vi "MotorControl_PWM+AO.vi"() -> ()   [LabVIEW 2015]
uses:
  <vilib>/Platform/TimedLoop/XDataNode/timing_clust.ctl
  <vilib>/Platform/TimedLoop/XDataNode/nitl_modes.ctl
  <vilib>/Platform/TimedLoop/XDataNode/wakeup.ctl
  <vilib>/rvi/FXPMathLib/FxpDiv/subVIs/nifxpmath_Div_SimConfig.ctl
  <vilib>/rvi/Emulation/niFpgaGetClockAttributes.vi
  <vilib>/rvi/Emulation/niFpgaSctlEmulationGetInTimedLoop.vi
  <vilib>/rvi/Emulation/niFpgaEmulationReportErrorSimple.vi
  <vilib>/rvi/FXPMathLib/FxpDiv/simVIs/DllFxpDivTemp_sub.vi
  GVEncoder.vi
  <vilib>/rvi/Emulation/niFpgaCriticalErrorInLSC.vi
  <vilib>/rvi/Emulation/niFpgaProcessEmulError.vi
  <vilib>/rvi/eio/common/nirviEmuTemplateMethod_errors.vi
  <vilib>/rvi/FXPMathLib/FxpMul/XNode/nifxpmath_Multiplier.xnode
  <vilib>/rvi/FXPMathLib/FxpDiv/XNode/nifxpmath_Div.xnode
  <vilib>/eio/EIONode/EIONode.xnode
  <vilib>/Platform/TimedLoop/XDataNode/XDataNode.xnode
  <vilib>/Platform/TimedLoop/XDataNode/XDNodeRunTimeDep.lvlib
  <vilib>/rvi/FXPMathLib/sim/FxpSim.dll
panel:
  out "ES_PRESSED":bool
  out "PWR_OK":bool
  in  "PWM (Hz/A)":fxp<+/-,32,16>=13.333328247070312 format="%#_21g"
  in  "EncdRst":bool[](array[boolean])=[FALSE, FALSE, FALSE, FALSE, FALSE, FALSE, FALSE, FALSE]
  out "PWM":fxp<+,16,8>[](array[numeric])
  in  "AmpCmd":sgl[](array[numeric])=[0.0, 0.0, 0.0, 0.0, 0.0, 0.0, 0.0, 0.0] format="%#.3f"
  in  "DisableWhenNotReady":bool
  in  "EnableMaster":bool
  out "Ready":bool[](array[boolean])
  in  "Enable":bool[](array[boolean])=[FALSE, FALSE, FALSE, FALSE, FALSE, FALSE, FALSE, FALSE]
  in  "EncoderCount":fxp<+,16,16>=500.0
  in  "2pi":fxp<+/-,32,10>=6.283185243606567 format="%#_39g"
  out "EncdAngle":sgl[](array[numeric]) format="%#.3f"
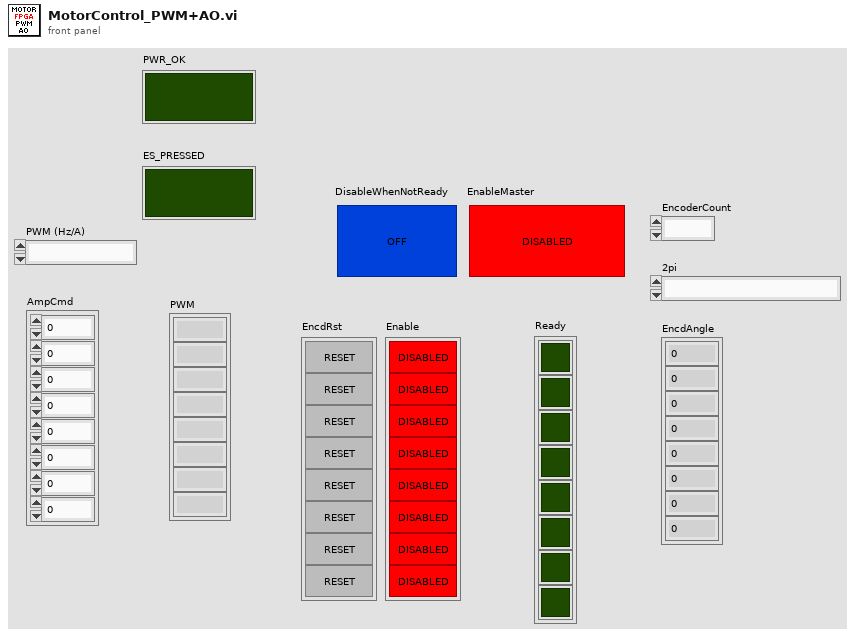
[diagram p1: front panel]
types:
  T1 = typedef "XDNodeRunTimeDep.lvlib/timing_clust.ctl" = cluster{"Expected End [f-1]":u64, "Actual End [f-1]":u64, "Finished Late? [f-1]":bool, "Expected End [i-1]":u64, "Actual End [i-1]":u64, "Finished Late? [i-1]":bool, "Expected Start [i]":u64, "Actual Start [i]":u64, "Expected Start [f]":u64, "Actual Start [f]":u64, "Source Name":string, "Structure Name":string, "Period":i64, "Deadline":i64, "Offset":i64, "Start":i64, "Priority":i32, "Timeout":i32, "Mode":T2, "Wakeup Reason":T3, "Error":errorcluster, "Source Type":string, "Secondary Source Type":string, "Global End Time":u64, "Global Start Time":u64, "Frame Duration":u64, "Iteration Duration":u64, "Assigned CPU":i32, "I/O Scan Engine Mode":u32}
  T2 = typedef "XDNodeRunTimeDep.lvlib/nitl_modes.ctl" = enum32{"No Change", "Process missed periods, maintain original phase", "Discard missed periods, maintain original phase", "Process missed periods, ignore original phase", "Discard missed periods, ignore original phase"}
  T3 = typedef "XDNodeRunTimeDep.lvlib/wakeup.ctl" = enum32{"Normal", "Aborted", "Asynchronous wakeup", "Timing source error", "Timed loop error", "Timeout"}
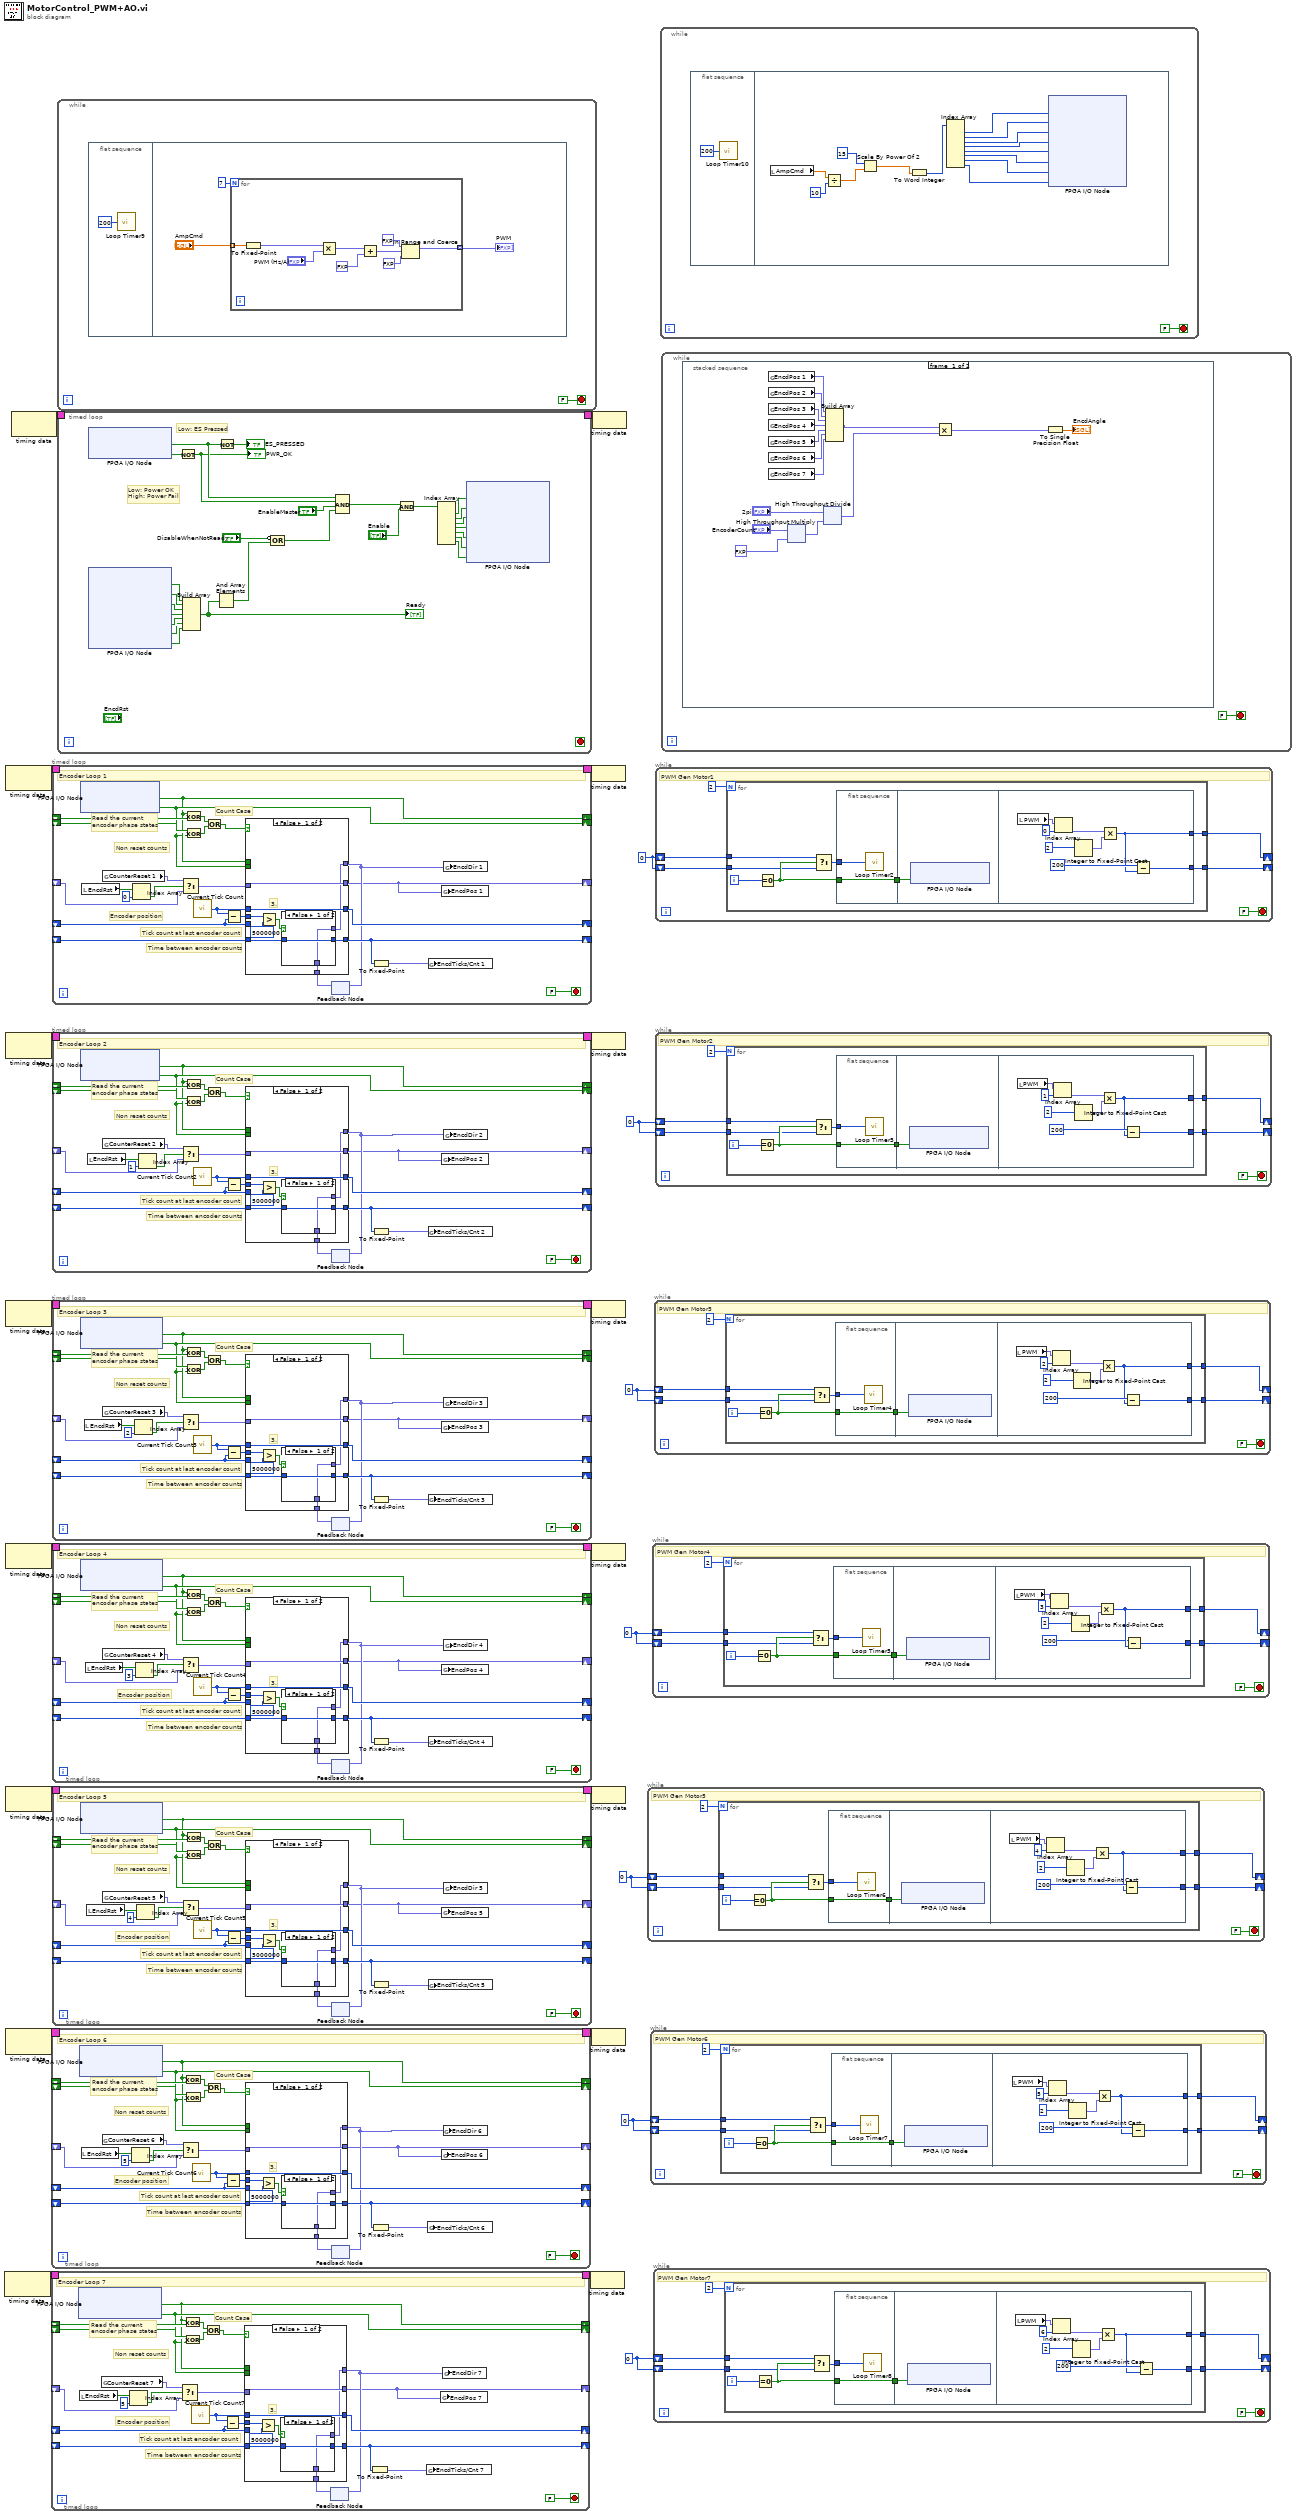
[diagram p0: block diagram]
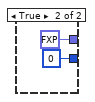
[diagram p2: hidden frame]
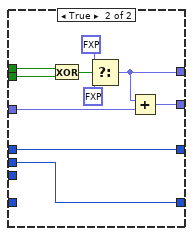
[diagram p3: hidden frame]
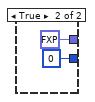
[diagram p4: hidden frame]
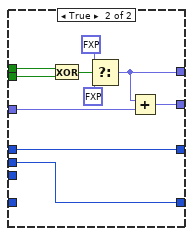
[diagram p5: hidden frame]
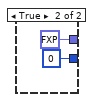
[diagram p6: hidden frame]
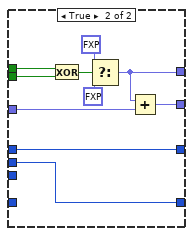
[diagram p7: hidden frame]
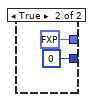
[diagram p8: hidden frame]
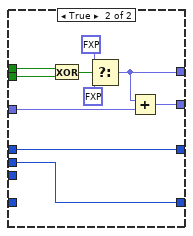
[diagram p9: hidden frame]
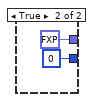
[diagram p10: hidden frame]
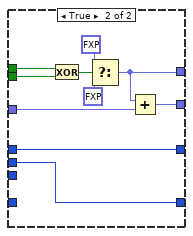
[diagram p11: hidden frame]
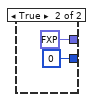
[diagram p12: hidden frame]
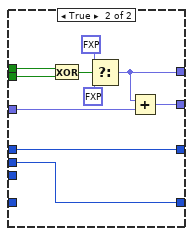
[diagram p13: hidden frame]
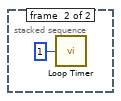
[diagram p14: hidden frame]
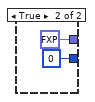
[diagram p15: hidden frame]
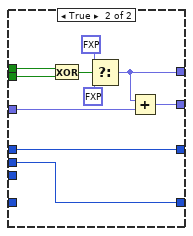
[diagram p16: hidden frame]
diagram:
  w1 = u32 0
  w2 = u32 0
  w3 = u32 0
  w4 = u32 0
  w5 = u32 0
  w6 = u32 0
  w7 = u32 0
  n1 = node-c288() -> (w11:T1)  [unwired: 1 in]
  n2 = node-c288() -> (w13:T1)  [unwired: 1 in]
  n3 = node-c288() -> (w23:T1)  [unwired: 1 in]
  n4 = node-c288() -> (w21:T1)  [unwired: 1 in]
  n5 = node-c288() -> (w19:T1)  [unwired: 1 in]
  n6 = node-c288() -> (w17:T1)  [unwired: 1 in]
  n7 = node-c288() -> (w15:T1)  [unwired: 1 in]
  n8 = node-c288() -> (w9:T1)  [unwired: 1 in]
  n9 = timed-loop {
    shift-right: [w41] -> _
    shift-left: _ -> [w47]
    shift-right: [w42] -> _
    shift-left: _ -> [w40]
    shift-right: [w28] -> _
    shift-left: _ -> [w46]
    shift-right: [w45] -> _
    shift-left: _ -> [w39]
    shift-right: [w32] -> _
    shift-left: _ -> [w44]
    timing: w11 -> [_]
    timing-out: [_] -> w10
    stop <- FALSE stop-if-true
    # "Count Case"
    # "Read the current\nencoder phase states"
    # "Non reset counts"
    # "Encoder position"
    # "Time between encoder counts"
    # "Tick count at last encoder count"
    # "Encoder Loop 7"
    n10 = xnode "FPGA I/O Node"() -> ("Connector1/DIO33"=w41:bool, "Connector1/DIO34"=w42:bool)  [unwired: 2 in, 2 out]
    n11 = local read "EncdRst"() -> (w26:bool[])
    n12 = global read "GVEncoder.vi" "CounterReset 7"() -> (w29:fxp<+/-,32,32>)
    n13 = Index Array(array=w26, index=5) -> (element=w24:bool)
    n14 = Select(t=w29, s=w24, f=w46) -> (s? t:f=w35:fxp<+/-,32,32>)
    n15 = Exclusive Or(1:w47, 2:w41) -> (0:w38:bool)
    n16 = Exclusive Or(1:w40, 2:w42) -> (0:w37:bool)
    n17 = call "Current Tick Count7"() -> ("Tick Count(Ticks)"=w33:u32)
    n18 = Or(x=w38, y=w37) -> (x .or. y?=w36:bool)
    n19 = Subtract(x=w33, y=w39) -> (x-y=w34:u32)
    n20 = feedback #1() -> (w31:fxp<+/-,2,2>)  [unwired: 1 in]
    n21 = case shown="False" w36 {
      tunnel: [w56 w64] -> w28
      tunnel: w35 -> [w56 w70]
      tunnel: [w50 w63] -> w45
      tunnel: w39 -> [w50 _]
      tunnel: [w53 w62] -> w32
      tunnel: w44 -> [w52 _]
      tunnel: w41 -> [_ w66]
      tunnel: w40 -> [_ w65]
      tunnel: w34 -> [w51 w62]
      tunnel: w33 -> [_ w63]
      tunnel: [w49 w61] -> w30
      tunnel: w31 -> [w48 _]
      frame False {
        # "3."
        n22 = Greater?(x=w51, y=u32 5000000 ("x")) -> (0:w54:bool)
        n23 = case shown="False" w54 {
          tunnel: [w58 u32 0 ("x")] -> w53
          tunnel: w52 -> [w58 _]
          tunnel: [w57 fxp<+/-,2,2> 0.0 ("16 bit")] -> w49
          tunnel: w48 -> [w57 _]
          frame False {
          }
          frame True {
          }
        }
      }
      frame True {
        n24 = Exclusive Or(1:w65, 2:w66) -> (0:w67:bool)
        n25 = Select(t=fxp<+,1,1> 1.0 ("16 bit"), s=w67, f=fxp<+/-,1,1> -1.0 ("16 bit")) -> (s? t:f=w61:fxp<+/-,2,2>)
        n26 = Add(x=w61, y=w70) -> (x+y=w64:fxp<+/-,32,32>)
      }
    }
    n27 = feedback-in #1(w30) -> ()
    n28 = To Fixed-Point(number=w32) -> (fixed-point=w27:fxp<+,32,32>)  [unwired: 1 in]
    n29 = global write "GVEncoder.vi" "EncdTicks/Cnt 7"(w27) -> ()
    n30 = global write "GVEncoder.vi" "EncdPos 7"(w28) -> ()
    n31 = global write "GVEncoder.vi" "EncdDir 7"(w30) -> ()
  }
  n32 = timed-loop {
    shift-right: [w90] -> _
    shift-left: _ -> [w96]
    shift-right: [w91] -> _
    shift-left: _ -> [w89]
    shift-right: [w77] -> _
    shift-left: _ -> [w95]
    shift-right: [w94] -> _
    shift-left: _ -> [w88]
    shift-right: [w81] -> _
    shift-left: _ -> [w93]
    timing: w13 -> [_]
    timing-out: [_] -> w12
    stop <- FALSE stop-if-true
    # "Count Case"
    # "Read the current\nencoder phase states"
    # "Non reset counts"
    # "Encoder position"
    # "Time between encoder counts"
    # "Tick count at last encoder count"
    # "Encoder Loop 6"
    n33 = xnode "FPGA I/O Node"() -> ("Connector1/DIO28"=w90:bool, "Connector1/DIO29"=w91:bool)  [unwired: 2 in, 2 out]
    n34 = local read "EncdRst"() -> (w74:bool[])
    n35 = global read "GVEncoder.vi" "CounterReset 6"() -> (w78:fxp<+/-,32,32>)
    n36 = Index Array(array=w74, index=5) -> (element=w73:bool)
    n37 = Select(t=w78, s=w73, f=w95) -> (s? t:f=w84:fxp<+/-,32,32>)
    n38 = Exclusive Or(1:w96, 2:w90) -> (0:w87:bool)
    n39 = Exclusive Or(1:w89, 2:w91) -> (0:w86:bool)
    n40 = call "Current Tick Count6"() -> ("Tick Count(Ticks)"=w82:u32)
    n41 = Or(x=w87, y=w86) -> (x .or. y?=w85:bool)
    n42 = Subtract(x=w82, y=w88) -> (x-y=w83:u32)
    n43 = feedback #2() -> (w80:fxp<+/-,2,2>)  [unwired: 1 in]
    n44 = case shown="False" w85 {
      tunnel: [w105 w113] -> w77
      tunnel: w84 -> [w105 w119]
      tunnel: [w99 w112] -> w94
      tunnel: w88 -> [w99 _]
      tunnel: [w102 w111] -> w81
      tunnel: w93 -> [w101 _]
      tunnel: w90 -> [_ w115]
      tunnel: w89 -> [_ w114]
      tunnel: w83 -> [w100 w111]
      tunnel: w82 -> [_ w112]
      tunnel: [w98 w110] -> w79
      tunnel: w80 -> [w97 _]
      frame False {
        # "3."
        n45 = Greater?(x=w100, y=u32 5000000 ("x")) -> (0:w103:bool)
        n46 = case shown="False" w103 {
          tunnel: [w107 u32 0 ("x")] -> w102
          tunnel: w101 -> [w107 _]
          tunnel: [w106 fxp<+/-,2,2> 0.0 ("16 bit")] -> w98
          tunnel: w97 -> [w106 _]
          frame False {
          }
          frame True {
          }
        }
      }
      frame True {
        n47 = Exclusive Or(1:w114, 2:w115) -> (0:w116:bool)
        n48 = Select(t=fxp<+,1,1> 1.0 ("16 bit"), s=w116, f=fxp<+/-,1,1> -1.0 ("16 bit")) -> (s? t:f=w110:fxp<+/-,2,2>)
        n49 = Add(x=w110, y=w119) -> (x+y=w113:fxp<+/-,32,32>)
      }
    }
    n50 = feedback-in #2(w79) -> ()
    n51 = To Fixed-Point(number=w81) -> (fixed-point=w76:fxp<+,32,32>)  [unwired: 1 in]
    n52 = global write "GVEncoder.vi" "EncdTicks/Cnt 6"(w76) -> ()
    n53 = global write "GVEncoder.vi" "EncdPos 6"(w77) -> ()
    n54 = global write "GVEncoder.vi" "EncdDir 6"(w79) -> ()
  }
  n55 = timed-loop {
    shift-right: [w139] -> _
    shift-left: _ -> [w145]
    shift-right: [w140] -> _
    shift-left: _ -> [w138]
    shift-right: [w126] -> _
    shift-left: _ -> [w144]
    shift-right: [w143] -> _
    shift-left: _ -> [w137]
    shift-right: [w130] -> _
    shift-left: _ -> [w142]
    timing: w23 -> [_]
    timing-out: [_] -> w22
    stop <- FALSE stop-if-true
    # "Count Case"
    # "Read the current\nencoder phase states"
    # "Non reset counts"
    # "Encoder position"
    # "Time between encoder counts"
    # "Tick count at last encoder count"
    # "Encoder Loop 1"
    n56 = xnode "FPGA I/O Node"() -> ("Connector1/DIO3"=w139:bool, "Connector1/DIO4"=w140:bool)  [unwired: 2 in, 2 out]
    n57 = local read "EncdRst"() -> (w124:bool[])
    n58 = global read "GVEncoder.vi" "CounterReset 1"() -> (w127:fxp<+/-,32,32>)
    n59 = Index Array(array=w124, index=0) -> (element=w122:bool)
    n60 = Select(t=w127, s=w122, f=w144) -> (s? t:f=w133:fxp<+/-,32,32>)
    n61 = Exclusive Or(1:w145, 2:w139) -> (0:w136:bool)
    n62 = Exclusive Or(1:w138, 2:w140) -> (0:w135:bool)
    n63 = call "Current Tick Count"() -> ("Tick Count(Ticks)"=w131:u32)
    n64 = Or(x=w136, y=w135) -> (x .or. y?=w134:bool)
    n65 = Subtract(x=w131, y=w137) -> (x-y=w132:u32)
    n66 = feedback #3() -> (w129:fxp<+/-,2,2>)  [unwired: 1 in]
    n67 = case shown="False" w134 {
      tunnel: [w154 w162] -> w126
      tunnel: w133 -> [w154 w168]
      tunnel: [w148 w161] -> w143
      tunnel: w137 -> [w148 _]
      tunnel: [w151 w160] -> w130
      tunnel: w142 -> [w150 _]
      tunnel: w139 -> [_ w164]
      tunnel: w138 -> [_ w163]
      tunnel: w132 -> [w149 w160]
      tunnel: w131 -> [_ w161]
      tunnel: [w147 w159] -> w128
      tunnel: w129 -> [w146 _]
      frame False {
        # "3."
        n68 = Greater?(x=w149, y=u32 5000000 ("x")) -> (0:w152:bool)
        n69 = case shown="False" w152 {
          tunnel: [w156 u32 0 ("x")] -> w151
          tunnel: w150 -> [w156 _]
          tunnel: [w155 fxp<+/-,2,2> 0.0 ("16 bit")] -> w147
          tunnel: w146 -> [w155 _]
          frame False {
          }
          frame True {
          }
        }
      }
      frame True {
        n70 = Exclusive Or(1:w163, 2:w164) -> (0:w165:bool)
        n71 = Select(t=fxp<+,1,1> 1.0 ("16 bit"), s=w165, f=fxp<+/-,1,1> -1.0 ("16 bit")) -> (s? t:f=w159:fxp<+/-,2,2>)
        n72 = Add(x=w159, y=w168) -> (x+y=w162:fxp<+/-,32,32>)
      }
    }
    n73 = feedback-in #3(w128) -> ()
    n74 = To Fixed-Point(number=w130) -> (fixed-point=w125:fxp<+,32,32>)  [unwired: 1 in]
    n75 = global write "GVEncoder.vi" "EncdTicks/Cnt 1"(w125) -> ()
    n76 = global write "GVEncoder.vi" "EncdPos 1"(w126) -> ()
    n77 = global write "GVEncoder.vi" "EncdDir 1"(w128) -> ()
  }
  n78 = timed-loop {
    shift-right: [w188] -> _
    shift-left: _ -> [w194]
    shift-right: [w189] -> _
    shift-left: _ -> [w187]
    shift-right: [w175] -> _
    shift-left: _ -> [w193]
    shift-right: [w192] -> _
    shift-left: _ -> [w186]
    shift-right: [w179] -> _
    shift-left: _ -> [w191]
    timing: w21 -> [_]
    timing-out: [_] -> w20
    stop <- FALSE stop-if-true
    # "Count Case"
    # "Read the current\nencoder phase states"
    # "Non reset counts"
    # "Time between encoder counts"
    # "Tick count at last encoder count"
    # "Encoder Loop 2"
    n79 = xnode "FPGA I/O Node"() -> ("Connector1/DIO8"=w188:bool, "Connector1/DIO9"=w189:bool)  [unwired: 2 in, 2 out]
    n80 = local read "EncdRst"() -> (w172:bool[])
    n81 = global read "GVEncoder.vi" "CounterReset 2"() -> (w176:fxp<+/-,32,32>)
    n82 = Index Array(array=w172, index=1) -> (element=w171:bool)
    n83 = Select(t=w176, s=w171, f=w193) -> (s? t:f=w182:fxp<+/-,32,32>)
    n84 = Exclusive Or(1:w194, 2:w188) -> (0:w185:bool)
    n85 = Exclusive Or(1:w187, 2:w189) -> (0:w184:bool)
    n86 = call "Current Tick Count2"() -> ("Tick Count(Ticks)"=w180:u32)
    n87 = Or(x=w185, y=w184) -> (x .or. y?=w183:bool)
    n88 = Subtract(x=w180, y=w186) -> (x-y=w181:u32)
    n89 = feedback #4() -> (w178:fxp<+/-,2,2>)  [unwired: 1 in]
    n90 = case shown="False" w183 {
      tunnel: [w203 w211] -> w175
      tunnel: w182 -> [w203 w217]
      tunnel: [w197 w210] -> w192
      tunnel: w186 -> [w197 _]
      tunnel: [w200 w209] -> w179
      tunnel: w191 -> [w199 _]
      tunnel: w188 -> [_ w213]
      tunnel: w187 -> [_ w212]
      tunnel: w181 -> [w198 w209]
      tunnel: w180 -> [_ w210]
      tunnel: [w196 w208] -> w177
      tunnel: w178 -> [w195 _]
      frame False {
        # "3."
        n91 = Greater?(x=w198, y=u32 5000000 ("x")) -> (0:w201:bool)
        n92 = case shown="False" w201 {
          tunnel: [w205 u32 0 ("x")] -> w200
          tunnel: w199 -> [w205 _]
          tunnel: [w204 fxp<+/-,2,2> 0.0 ("16 bit")] -> w196
          tunnel: w195 -> [w204 _]
          frame False {
          }
          frame True {
          }
        }
      }
      frame True {
        n93 = Exclusive Or(1:w212, 2:w213) -> (0:w214:bool)
        n94 = Select(t=fxp<+,1,1> 1.0 ("16 bit"), s=w214, f=fxp<+/-,1,1> -1.0 ("16 bit")) -> (s? t:f=w208:fxp<+/-,2,2>)
        n95 = Add(x=w208, y=w217) -> (x+y=w211:fxp<+/-,32,32>)
      }
    }
    n96 = feedback-in #4(w177) -> ()
    n97 = To Fixed-Point(number=w179) -> (fixed-point=w174:fxp<+,32,32>)  [unwired: 1 in]
    n98 = global write "GVEncoder.vi" "EncdTicks/Cnt 2"(w174) -> ()
    n99 = global write "GVEncoder.vi" "EncdPos 2"(w175) -> ()
    n100 = global write "GVEncoder.vi" "EncdDir 2"(w177) -> ()
  }
  n101 = timed-loop {
    shift-right: [w237] -> _
    shift-left: _ -> [w243]
    shift-right: [w238] -> _
    shift-left: _ -> [w236]
    shift-right: [w224] -> _
    shift-left: _ -> [w242]
    shift-right: [w241] -> _
    shift-left: _ -> [w235]
    shift-right: [w228] -> _
    shift-left: _ -> [w240]
    timing: w19 -> [_]
    timing-out: [_] -> w18
    stop <- FALSE stop-if-true
    # "Count Case"
    # "Read the current\nencoder phase states"
    # "Non reset counts"
    # "Time between encoder counts"
    # "Tick count at last encoder count"
    # "Encoder Loop 3"
    n102 = xnode "FPGA I/O Node"() -> ("Connector1/DIO13"=w237:bool, "Connector1/DIO14"=w238:bool)  [unwired: 2 in, 2 out]
    n103 = local read "EncdRst"() -> (w222:bool[])
    n104 = global read "GVEncoder.vi" "CounterReset 3"() -> (w225:fxp<+/-,32,32>)
    n105 = Index Array(array=w222, index=2) -> (element=w220:bool)
    n106 = Select(t=w225, s=w220, f=w242) -> (s? t:f=w231:fxp<+/-,32,32>)
    n107 = Exclusive Or(1:w243, 2:w237) -> (0:w234:bool)
    n108 = Exclusive Or(1:w236, 2:w238) -> (0:w233:bool)
    n109 = call "Current Tick Count3"() -> ("Tick Count(Ticks)"=w229:u32)
    n110 = Or(x=w234, y=w233) -> (x .or. y?=w232:bool)
    n111 = Subtract(x=w229, y=w235) -> (x-y=w230:u32)
    n112 = feedback #5() -> (w227:fxp<+/-,2,2>)  [unwired: 1 in]
    n113 = case shown="False" w232 {
      tunnel: [w252 w260] -> w224
      tunnel: w231 -> [w252 w266]
      tunnel: [w246 w259] -> w241
      tunnel: w235 -> [w246 _]
      tunnel: [w249 w258] -> w228
      tunnel: w240 -> [w248 _]
      tunnel: w237 -> [_ w262]
      tunnel: w236 -> [_ w261]
      tunnel: w230 -> [w247 w258]
      tunnel: w229 -> [_ w259]
      tunnel: [w245 w257] -> w226
      tunnel: w227 -> [w244 _]
      frame False {
        # "3."
        n114 = Greater?(x=w247, y=u32 5000000 ("x")) -> (0:w250:bool)
        n115 = case shown="False" w250 {
          tunnel: [w254 u32 0 ("x")] -> w249
          tunnel: w248 -> [w254 _]
          tunnel: [w253 fxp<+/-,2,2> 0.0 ("16 bit")] -> w245
          tunnel: w244 -> [w253 _]
          frame False {
          }
          frame True {
          }
        }
      }
      frame True {
        n116 = Exclusive Or(1:w261, 2:w262) -> (0:w263:bool)
        n117 = Select(t=fxp<+,1,1> 1.0 ("16 bit"), s=w263, f=fxp<+/-,1,1> -1.0 ("16 bit")) -> (s? t:f=w257:fxp<+/-,2,2>)
        n118 = Add(x=w257, y=w266) -> (x+y=w260:fxp<+/-,32,32>)
      }
    }
    n119 = feedback-in #5(w226) -> ()
    n120 = To Fixed-Point(number=w228) -> (fixed-point=w223:fxp<+,32,32>)  [unwired: 1 in]
    n121 = global write "GVEncoder.vi" "EncdTicks/Cnt 3"(w223) -> ()
    n122 = global write "GVEncoder.vi" "EncdPos 3"(w224) -> ()
    n123 = global write "GVEncoder.vi" "EncdDir 3"(w226) -> ()
  }
  n124 = timed-loop {
    shift-right: [w286] -> _
    shift-left: _ -> [w292]
    shift-right: [w287] -> _
    shift-left: _ -> [w285]
    shift-right: [w273] -> _
    shift-left: _ -> [w291]
    shift-right: [w290] -> _
    shift-left: _ -> [w284]
    shift-right: [w277] -> _
    shift-left: _ -> [w289]
    timing: w17 -> [_]
    timing-out: [_] -> w16
    stop <- FALSE stop-if-true
    # "Count Case"
    # "Read the current\nencoder phase states"
    # "Non reset counts"
    # "Encoder position"
    # "Time between encoder counts"
    # "Tick count at last encoder count"
    # "Encoder Loop 4"
    n125 = xnode "FPGA I/O Node"() -> ("Connector1/DIO18"=w286:bool, "Connector1/DIO19"=w287:bool)  [unwired: 2 in, 2 out]
    n126 = local read "EncdRst"() -> (w270:bool[])
    n127 = global read "GVEncoder.vi" "CounterReset 4"() -> (w274:fxp<+/-,32,32>)
    n128 = Index Array(array=w270, index=3) -> (element=w269:bool)
    n129 = Select(t=w274, s=w269, f=w291) -> (s? t:f=w280:fxp<+/-,32,32>)
    n130 = Exclusive Or(1:w292, 2:w286) -> (0:w283:bool)
    n131 = Exclusive Or(1:w285, 2:w287) -> (0:w282:bool)
    n132 = call "Current Tick Count4"() -> ("Tick Count(Ticks)"=w278:u32)
    n133 = Or(x=w283, y=w282) -> (x .or. y?=w281:bool)
    n134 = Subtract(x=w278, y=w284) -> (x-y=w279:u32)
    n135 = feedback #6() -> (w276:fxp<+/-,2,2>)  [unwired: 1 in]
    n136 = case shown="False" w281 {
      tunnel: [w301 w309] -> w273
      tunnel: w280 -> [w301 w315]
      tunnel: [w295 w308] -> w290
      tunnel: w284 -> [w295 _]
      tunnel: [w298 w307] -> w277
      tunnel: w289 -> [w297 _]
      tunnel: w286 -> [_ w311]
      tunnel: w285 -> [_ w310]
      tunnel: w279 -> [w296 w307]
      tunnel: w278 -> [_ w308]
      tunnel: [w294 w306] -> w275
      tunnel: w276 -> [w293 _]
      frame False {
        # "3."
        n137 = Greater?(x=w296, y=u32 5000000 ("x")) -> (0:w299:bool)
        n138 = case shown="False" w299 {
          tunnel: [w303 u32 0 ("x")] -> w298
          tunnel: w297 -> [w303 _]
          tunnel: [w302 fxp<+/-,2,2> 0.0 ("16 bit")] -> w294
          tunnel: w293 -> [w302 _]
          frame False {
          }
          frame True {
          }
        }
      }
      frame True {
        n139 = Exclusive Or(1:w310, 2:w311) -> (0:w312:bool)
        n140 = Select(t=fxp<+,1,1> 1.0 ("16 bit"), s=w312, f=fxp<+/-,1,1> -1.0 ("16 bit")) -> (s? t:f=w306:fxp<+/-,2,2>)
        n141 = Add(x=w306, y=w315) -> (x+y=w309:fxp<+/-,32,32>)
      }
    }
    n142 = feedback-in #6(w275) -> ()
    n143 = To Fixed-Point(number=w277) -> (fixed-point=w272:fxp<+,32,32>)  [unwired: 1 in]
    n144 = global write "GVEncoder.vi" "EncdTicks/Cnt 4"(w272) -> ()
    n145 = global write "GVEncoder.vi" "EncdPos 4"(w273) -> ()
    n146 = global write "GVEncoder.vi" "EncdDir 4"(w275) -> ()
  }
  n147 = timed-loop {
    shift-right: [w335] -> _
    shift-left: _ -> [w341]
    shift-right: [w336] -> _
    shift-left: _ -> [w334]
    shift-right: [w322] -> _
    shift-left: _ -> [w340]
    shift-right: [w339] -> _
    shift-left: _ -> [w333]
    shift-right: [w326] -> _
    shift-left: _ -> [w338]
    timing: w15 -> [_]
    timing-out: [_] -> w14
    stop <- FALSE stop-if-true
    # "Count Case"
    # "Read the current\nencoder phase states"
    # "Non reset counts"
    # "Encoder position"
    # "Time between encoder counts"
    # "Tick count at last encoder count"
    # "Encoder Loop 5"
    n148 = xnode "FPGA I/O Node"() -> ("Connector1/DIO23"=w335:bool, "Connector1/DIO24"=w336:bool)  [unwired: 2 in, 2 out]
    n149 = local read "EncdRst"() -> (w320:bool[])
    n150 = global read "GVEncoder.vi" "CounterReset 5"() -> (w323:fxp<+/-,32,32>)
    n151 = Index Array(array=w320, index=4) -> (element=w318:bool)
    n152 = Select(t=w323, s=w318, f=w340) -> (s? t:f=w329:fxp<+/-,32,32>)
    n153 = Exclusive Or(1:w341, 2:w335) -> (0:w332:bool)
    n154 = Exclusive Or(1:w334, 2:w336) -> (0:w331:bool)
    n155 = call "Current Tick Count5"() -> ("Tick Count(Ticks)"=w327:u32)
    n156 = Or(x=w332, y=w331) -> (x .or. y?=w330:bool)
    n157 = Subtract(x=w327, y=w333) -> (x-y=w328:u32)
    n158 = feedback #7() -> (w325:fxp<+/-,2,2>)  [unwired: 1 in]
    n159 = case shown="False" w330 {
      tunnel: [w350 w358] -> w322
      tunnel: w329 -> [w350 w364]
      tunnel: [w344 w357] -> w339
      tunnel: w333 -> [w344 _]
      tunnel: [w347 w356] -> w326
      tunnel: w338 -> [w346 _]
      tunnel: w335 -> [_ w360]
      tunnel: w334 -> [_ w359]
      tunnel: w328 -> [w345 w356]
      tunnel: w327 -> [_ w357]
      tunnel: [w343 w355] -> w324
      tunnel: w325 -> [w342 _]
      frame False {
        # "3."
        n160 = Greater?(x=w345, y=u32 5000000 ("x")) -> (0:w348:bool)
        n161 = case shown="False" w348 {
          tunnel: [w352 u32 0 ("x")] -> w347
          tunnel: w346 -> [w352 _]
          tunnel: [w351 fxp<+/-,2,2> 0.0 ("16 bit")] -> w343
          tunnel: w342 -> [w351 _]
          frame False {
          }
          frame True {
          }
        }
      }
      frame True {
        n162 = Exclusive Or(1:w359, 2:w360) -> (0:w361:bool)
        n163 = Select(t=fxp<+,1,1> 1.0 ("16 bit"), s=w361, f=fxp<+/-,1,1> -1.0 ("16 bit")) -> (s? t:f=w355:fxp<+/-,2,2>)
        n164 = Add(x=w355, y=w364) -> (x+y=w358:fxp<+/-,32,32>)
      }
    }
    n165 = feedback-in #7(w324) -> ()
    n166 = To Fixed-Point(number=w326) -> (fixed-point=w321:fxp<+,32,32>)  [unwired: 1 in]
    n167 = global write "GVEncoder.vi" "EncdTicks/Cnt 5"(w321) -> ()
    n168 = global write "GVEncoder.vi" "EncdPos 5"(w322) -> ()
    n169 = global write "GVEncoder.vi" "EncdDir 5"(w324) -> ()
  }
  n170 = timed-loop {
    timing: w9 -> [_]
    timing-out: [_] -> w8
    stop <- _ stop-if-true
    # "Low: ES Pressed"
    # "Low: Power OK\nHigh: Power Fail"
    n171 = xnode "FPGA I/O Node"() -> ("Connector1/DIO37"=w371:bool, "Connector1/DIO36"=w370:bool)  [unwired: 2 in, 2 out]
    n172 = xnode "FPGA I/O Node"() -> ("Connector1/DIO2"=w390:bool, "Connector1/DIO7"=w389:bool, "Connector1/DIO12"=w388:bool, "Connector1/DIO17"=w387:bool, "Connector1/DIO22"=w386:bool, "Connector1/DIO27"=w385:bool, "Connector1/DIO32"=w384:bool)  [unwired: 7 in, 7 out]
    n173 = Not(x=w370) -> (.not. x?=w368:bool)
    "PWR_OK" <- w368
    n174 = Build Array(w390, w389, w388, w387, w386, w385, w384) -> (w367:bool[])
    "Ready" <- w367
    n175 = And Array Elements(Boolean array=w367) -> (logical AND=w382:bool)
    n176 = Not(x=w371) -> (.not. x?=→"ES_PRESSED":bool)
    n177 = Compound Arithmetic op=OR(invert "DisableWhenNotReady", w382) -> (w373:bool)
    n178 = Compound Arithmetic op=AND(w371, w368, "EnableMaster", w373) -> (w374:bool)
    n179 = And(x=w374, y="Enable") -> (x .and. y?=w391:bool[])
    n180 = Index Array(array=w391) -> (element #1=w381:bool, element #2=w380:bool, element #3=w379:bool, element #4=w378:bool, element #5=w377:bool, element #6=w376:bool, element #7=w375:bool)  [unwired: 7 in]
    n181 = xnode "FPGA I/O Node"("Connector1/DIO1"=w381, "Connector1/DIO6"=w380, "Connector1/DIO11"=w379, "Connector1/DIO16"=w378, "Connector1/DIO21"=w377, "Connector1/DIO26"=w376, "Connector1/DIO31"=w375) -> ()  [unwired: 7 in, 7 out]
  }
  n182 = while {
    stop <- FALSE stop-if-true
    n183 = flat-sequence {
      frame #0 {
        n184 = call "Loop Timer9"("Count(uSec)"=u32 200) -> ()  [unwired: 1 out]
      }
      frame #1 {
        n185 = for {
          N: 7 -> [_]
          tunnel: "AmpCmd" -> [w408] mode=indexing
          tunnel: [w400] -> w397 mode=indexing
          n186 = To Fixed-Point(number=w408) -> (fixed-point=w407:fxp<+/-,32,16>)  [unwired: 1 in]
          n187 = Multiply(x=w407, y="PWM (Hz/A)") -> (x*y=w405:fxp<+/-,16,8>)
          n188 = Add(x=w405, y=fxp<+,16,8> 50.0) -> (x+y=w401:fxp<+,16,8>)
          n189 = In Range and Coerce(upper limit=fxp<+,16,8> 90.0 ("y"), x=w401, lower limit=fxp<+,16,8> 10.0 ("y")) -> (coerced(x)=w400:fxp<+,16,8>)  [unwired: 1 out]
        }
        "PWM" <- w397
      }
    }
  }
  n190 = node-c288(w10) -> ()
  n191 = node-c288(w12) -> ()
  n192 = node-c288(w22) -> ()
  n193 = node-c288(w20) -> ()
  n194 = node-c288(w18) -> ()
  n195 = node-c288(w16) -> ()
  n196 = node-c288(w14) -> ()
  n197 = node-c288(w8) -> ()
  n198 = while {
    shift-right: [w410] -> _
    shift-left: w4 -> [w413]
    shift-right: [w411] -> _
    shift-left: w4 -> [w412]
    stop <- FALSE stop-if-true
    # "PWM Gen Motor5"
    n199 = for {
      N: 2 -> [_]
      tunnel: w413 -> [w417]
      tunnel: w412 -> [w418]
      tunnel: [w416] -> w411
      tunnel: [w415] -> w410
      i -> [w422]
      n200 = Equal To 0?(x=w422) -> (x = 0?=w419:bool)
      n201 = Select(t=w417, s=w419, f=w418) -> (s? t:f=w421:u32)
      n202 = flat-sequence {
        tunnel: w421 -> [w423]
        tunnel: [w424] -> w420
        tunnel: w419 -> [w424]
        tunnel: w420 -> [w425]
        tunnel: [w433] -> w416
        tunnel: [w426] -> w415
        frame #0 {
          n203 = call "Loop Timer6"("Count(uSec)"=w423) -> ()  [unwired: 1 out]
        }
        frame #1 {
          n204 = xnode "FPGA I/O Node"("Connector1/DIO20"=w425) -> ()  [unwired: 1 in, 1 out]
        }
        frame #2 {
          n205 = local read "PWM"() -> (w430:fxp<+,16,8>[])
          n206 = Index Array(array=w430, index=4) -> (element=w429:fxp<+,16,8>)
          n207 = Integer to Fixed-Point Cast(integer=u32 2) -> (fixed-point=w431:fxp<+,32,32>)  [unwired: 1 in]
          n208 = Multiply(x=w429, y=w431) -> (x*y=w426:u32)
          n209 = Subtract(x=u32 200, y=w426) -> (x-y=w433:u32)
        }
      }
    }
  }
  n210 = while {
    shift-right: [w435] -> _
    shift-left: w3 -> [w438]
    shift-right: [w436] -> _
    shift-left: w3 -> [w437]
    stop <- FALSE stop-if-true
    # "PWM Gen Motor6"
    n211 = for {
      N: 2 -> [_]
      tunnel: w438 -> [w442]
      tunnel: w437 -> [w443]
      tunnel: [w441] -> w436
      tunnel: [w440] -> w435
      i -> [w447]
      n212 = Equal To 0?(x=w447) -> (x = 0?=w444:bool)
      n213 = Select(t=w442, s=w444, f=w443) -> (s? t:f=w446:u32)
      n214 = flat-sequence {
        tunnel: w446 -> [w448]
        tunnel: [w449] -> w445
        tunnel: w444 -> [w449]
        tunnel: w445 -> [w450]
        tunnel: [w458] -> w441
        tunnel: [w451] -> w440
        frame #0 {
          n215 = call "Loop Timer7"("Count(uSec)"=w448) -> ()  [unwired: 1 out]
        }
        frame #1 {
          n216 = xnode "FPGA I/O Node"("Connector1/DIO25"=w450) -> ()  [unwired: 1 in, 1 out]
        }
        frame #2 {
          n217 = local read "PWM"() -> (w455:fxp<+,16,8>[])
          n218 = Index Array(array=w455, index=5) -> (element=w454:fxp<+,16,8>)
          n219 = Integer to Fixed-Point Cast(integer=u32 2) -> (fixed-point=w456:fxp<+,32,32>)  [unwired: 1 in]
          n220 = Multiply(x=w454, y=w456) -> (x*y=w451:u32)
          n221 = Subtract(x=u32 200, y=w451) -> (x-y=w458:u32)
        }
      }
    }
  }
  n222 = while {
    shift-right: [w460] -> _
    shift-left: w5 -> [w463]
    shift-right: [w461] -> _
    shift-left: w5 -> [w462]
    stop <- FALSE stop-if-true
    # "PWM Gen Motor4"
    n223 = for {
      N: 2 -> [_]
      tunnel: w463 -> [w467]
      tunnel: w462 -> [w468]
      tunnel: [w466] -> w461
      tunnel: [w465] -> w460
      i -> [w472]
      n224 = Equal To 0?(x=w472) -> (x = 0?=w469:bool)
      n225 = Select(t=w467, s=w469, f=w468) -> (s? t:f=w471:u32)
      n226 = flat-sequence {
        tunnel: w471 -> [w473]
        tunnel: [w474] -> w470
        tunnel: w469 -> [w474]
        tunnel: w470 -> [w475]
        tunnel: [w483] -> w466
        tunnel: [w477] -> w465
        frame #0 {
          n227 = call "Loop Timer5"("Count(uSec)"=w473) -> ()  [unwired: 1 out]
        }
        frame #1 {
          n228 = xnode "FPGA I/O Node"("Connector1/DIO15"=w475) -> ()  [unwired: 1 in, 1 out]
        }
        frame #2 {
          n229 = local read "PWM"() -> (w480:fxp<+,16,8>[])
          n230 = Index Array(array=w480, index=3) -> (element=w479:fxp<+,16,8>)
          n231 = Integer to Fixed-Point Cast(integer=u32 2) -> (fixed-point=w481:fxp<+,32,32>)  [unwired: 1 in]
          n232 = Multiply(x=w479, y=w481) -> (x*y=w477:u32)
          n233 = Subtract(x=u32 200, y=w477) -> (x-y=w483:u32)
        }
      }
    }
  }
  n234 = while {
    shift-right: [w485] -> _
    shift-left: w2 -> [w488]
    shift-right: [w486] -> _
    shift-left: w2 -> [w487]
    stop <- FALSE stop-if-true
    # "PWM Gen Motor7"
    n235 = for {
      N: 2 -> [_]
      tunnel: w488 -> [w492]
      tunnel: w487 -> [w493]
      tunnel: [w491] -> w486
      tunnel: [w490] -> w485
      i -> [w497]
      n236 = Equal To 0?(x=w497) -> (x = 0?=w494:bool)
      n237 = Select(t=w492, s=w494, f=w493) -> (s? t:f=w496:u32)
      n238 = flat-sequence {
        tunnel: w496 -> [w498]
        tunnel: [w499] -> w495
        tunnel: w494 -> [w499]
        tunnel: w495 -> [w500]
        tunnel: [w508] -> w491
        tunnel: [w501] -> w490
        frame #0 {
          n239 = call "Loop Timer8"("Count(uSec)"=w498) -> ()  [unwired: 1 out]
        }
        frame #1 {
          n240 = xnode "FPGA I/O Node"("Connector1/DIO30"=w500) -> ()  [unwired: 1 in, 1 out]
        }
        frame #2 {
          n241 = local read "PWM"() -> (w505:fxp<+,16,8>[])
          n242 = Index Array(array=w505, index=6) -> (element=w504:fxp<+,16,8>)
          n243 = Integer to Fixed-Point Cast(integer=u32 2) -> (fixed-point=w506:fxp<+,32,32>)  [unwired: 1 in]
          n244 = Multiply(x=w504, y=w506) -> (x*y=w501:u32)
          n245 = Subtract(x=u32 200, y=w501) -> (x-y=w508:u32)
        }
      }
    }
  }
  n246 = while {
    shift-right: [w510] -> _
    shift-left: w6 -> [w513]
    shift-right: [w511] -> _
    shift-left: w6 -> [w512]
    stop <- FALSE stop-if-true
    # "PWM Gen Motor3"
    n247 = for {
      N: 2 -> [_]
      tunnel: w513 -> [w517]
      tunnel: w512 -> [w518]
      tunnel: [w516] -> w511
      tunnel: [w515] -> w510
      i -> [w522]
      n248 = Equal To 0?(x=w522) -> (x = 0?=w519:bool)
      n249 = Select(t=w517, s=w519, f=w518) -> (s? t:f=w521:u32)
      n250 = flat-sequence {
        tunnel: w521 -> [w523]
        tunnel: [w524] -> w520
        tunnel: w519 -> [w524]
        tunnel: w520 -> [w525]
        tunnel: [w533] -> w516
        tunnel: [w526] -> w515
        frame #0 {
          n251 = call "Loop Timer4"("Count(uSec)"=w523) -> ()  [unwired: 1 out]
        }
        frame #1 {
          n252 = xnode "FPGA I/O Node"("Connector1/DIO10"=w525) -> ()  [unwired: 1 in, 1 out]
        }
        frame #2 {
          n253 = local read "PWM"() -> (w530:fxp<+,16,8>[])
          n254 = Index Array(array=w530, index=2) -> (element=w529:fxp<+,16,8>)
          n255 = Integer to Fixed-Point Cast(integer=u32 2) -> (fixed-point=w531:fxp<+,32,32>)  [unwired: 1 in]
          n256 = Multiply(x=w529, y=w531) -> (x*y=w526:u32)
          n257 = Subtract(x=u32 200, y=w526) -> (x-y=w533:u32)
        }
      }
    }
  }
  n258 = while {
    shift-right: [w535] -> _
    shift-left: w7 -> [w538]
    shift-right: [w536] -> _
    shift-left: w7 -> [w537]
    stop <- FALSE stop-if-true
    # "PWM Gen Motor2"
    n259 = for {
      N: 2 -> [_]
      tunnel: w538 -> [w542]
      tunnel: w537 -> [w543]
      tunnel: [w541] -> w536
      tunnel: [w540] -> w535
      i -> [w547]
      n260 = Equal To 0?(x=w547) -> (x = 0?=w544:bool)
      n261 = Select(t=w542, s=w544, f=w543) -> (s? t:f=w546:u32)
      n262 = flat-sequence {
        tunnel: w546 -> [w548]
        tunnel: [w549] -> w545
        tunnel: w544 -> [w549]
        tunnel: w545 -> [w550]
        tunnel: [w558] -> w541
        tunnel: [w551] -> w540
        frame #0 {
          n263 = call "Loop Timer3"("Count(uSec)"=w548) -> ()  [unwired: 1 out]
        }
        frame #1 {
          n264 = xnode "FPGA I/O Node"("Connector1/DIO5"=w550) -> ()  [unwired: 1 in, 1 out]
        }
        frame #2 {
          n265 = local read "PWM"() -> (w555:fxp<+,16,8>[])
          n266 = Index Array(array=w555, index=1) -> (element=w554:fxp<+,16,8>)
          n267 = Integer to Fixed-Point Cast(integer=u32 2) -> (fixed-point=w556:fxp<+,32,32>)  [unwired: 1 in]
          n268 = Multiply(x=w554, y=w556) -> (x*y=w551:u32)
          n269 = Subtract(x=u32 200, y=w551) -> (x-y=w558:u32)
        }
      }
    }
  }
  n270 = while {
    shift-right: [w560] -> _
    shift-left: w1 -> [w563]
    shift-right: [w561] -> _
    shift-left: w1 -> [w562]
    stop <- FALSE stop-if-true
    # "PWM Gen Motor1"
    n271 = for {
      N: 2 -> [_]
      tunnel: w563 -> [w567]
      tunnel: w562 -> [w568]
      tunnel: [w566] -> w561
      tunnel: [w565] -> w560
      i -> [w572]
      n272 = Equal To 0?(x=w572) -> (x = 0?=w569:bool)
      n273 = Select(t=w567, s=w569, f=w568) -> (s? t:f=w571:u32)
      n274 = flat-sequence {
        tunnel: w571 -> [w573]
        tunnel: [w574] -> w570
        tunnel: w569 -> [w574]
        tunnel: w570 -> [w575]
        tunnel: [w583] -> w566
        tunnel: [w576] -> w565
        frame #0 {
          n275 = call "Loop Timer2"("Count(uSec)"=w573) -> ()  [unwired: 1 out]
        }
        frame #1 {
          n276 = xnode "FPGA I/O Node"("Connector1/DIO0"=w575) -> ()  [unwired: 1 in, 1 out]
        }
        frame #2 {
          n277 = local read "PWM"() -> (w580:fxp<+,16,8>[])
          n278 = Index Array(array=w580, index=0) -> (element=w579:fxp<+,16,8>)
          n279 = Integer to Fixed-Point Cast(integer=u32 2) -> (fixed-point=w581:fxp<+,32,32>)  [unwired: 1 in]
          n280 = Multiply(x=w579, y=w581) -> (x*y=w576:u32)
          n281 = Subtract(x=u32 200, y=w576) -> (x-y=w583:u32)
        }
      }
    }
  }
  n282 = while {
    stop <- FALSE stop-if-true
    n283 = flat-sequence {
      frame #0 {
        n284 = call "Loop Timer10"("Count(uSec)"=u32 200) -> ()  [unwired: 1 out]
      }
      frame #1 {
        n285 = local read "AmpCmd"() -> (w599:sgl[])
        n286 = Divide(x=w599, y=i16 10) -> (x/y=w597:sgl[])
        n287 = Scale By Power Of 2(n=i16 15, x=w597) -> (x*2^n=w595:sgl[])
        n288 = To Word Integer(number=w595) -> (16bit integer=w594:i16[])
        n289 = Index Array(array=w594) -> (element #1=w593:i16, element #2=w592:i16, element #3=w591:i16, element #4=w590:i16, element #5=w589:i16, element #6=w588:i16, element #7=w587:i16, element #8=w586:i16)  [unwired: 8 in]
        n290 = xnode "FPGA I/O Node"("Connector0/AO0"=w593, "Connector0/AO1"=w592, "Connector0/AO2"=w591, "Connector0/AO3"=w590, "Connector0/AO4"=w589, "Connector0/AO5"=w588, "Connector0/AO6"=w587, "Connector0/AO7"=w586) -> ()  [unwired: 8 in, 8 out]
      }
    }
  }
  n291 = while {
    stop <- FALSE stop-if-true
    n292 = stacked-sequence {
      frame #0 {
        n293 = global read "GVEncoder.vi" "EncdPos 1"() -> (w614:fxp<+/-,32,32>)
        n294 = global read "GVEncoder.vi" "EncdPos 2"() -> (w613:fxp<+/-,32,32>)
        n295 = global read "GVEncoder.vi" "EncdPos 3"() -> (w612:fxp<+/-,32,32>)
        n296 = global read "GVEncoder.vi" "EncdPos 4"() -> (w606:fxp<+/-,32,32>)
        n297 = global read "GVEncoder.vi" "EncdPos 5"() -> (w605:fxp<+/-,32,32>)
        n298 = global read "GVEncoder.vi" "EncdPos 6"() -> (w604:fxp<+/-,32,32>)
        n299 = global read "GVEncoder.vi" "EncdPos 7"() -> (w603:fxp<+/-,32,32>)
        n300 = xnode ("High Throughput Multiply")("x"="EncoderCount", "y"=fxp<+,4,4> 4.0) -> ("x*y"=w608:fxp<+,16,16>)
        n301 = xnode "High Throughput Divide"("x"="2pi", "y"=w608) -> ("x/y"=w601:fxp<+/-,32,4>)
        n302 = Build Array(w614, w613, w612, w606, w605, w604, w603) -> (w602:fxp<+/-,32,32>[])
        n303 = Multiply(x=w602, y=w601) -> (x*y=w610:fxp<+/-,32,16>[])
        n304 = To Single Precision Float(number=w610) -> (single precision float=→"EncdAngle":sgl[])
      }
      frame #1 {
        n305 = call "Loop Timer"("Count(uSec)"=u32 1) -> ()  [unwired: 1 out]
      }
    }
  }
